vi "SVT Exp Avg Sound Level (1 Ch).vi"(6 "restart averaging (F)":bool, 8 "error in (no error)":errorcluster, 9 "time constant [ms]":dbl=125.0 format="%.2f", 10 "exponential mode":enum16{"Slow", "Fast", "Impulse", "Custom"}(ring)=enum."Fast", 11 "scaled signal [EU]":waveform(dbl)) -> (0 "error out":errorcluster, 1 "actual time constant [ms]":dbl=nan format="%.2f", 2 "unit label":string, 3 "exp avg sound level [dB EU]":waveform(dbl), 4 "maximum sound level [dB EU]":dbl=nan format="%.2f")   [LabVIEW 2017]
doc: "Computes the exponential averaged sound level of <B>scaled signal [EU]</B> based on <B>exponential mode</B> and returns the sound level for the signal in <B>exp avg sound level [dB EU]</B>. The SVL Exp Avg Sound Level VI returns the exponential average sound level computed after each individual sample of the time record. You can use this polymorphic VI to compute the exponential averaged sound level for a single channel or for N channels. The data type you wire to the <B>scaled signal [EU]</B> input determines the polymorphic instance to use."
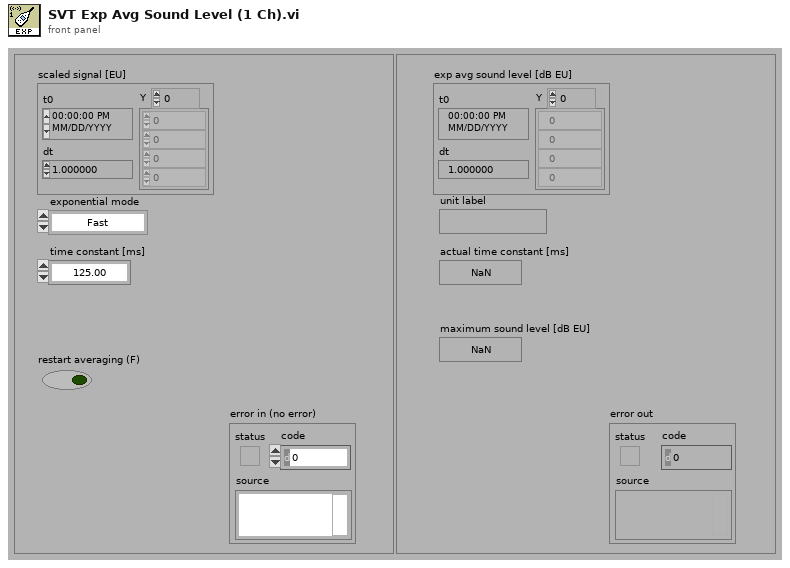
[diagram p1: front panel]
types:
  T1 = enum16{"RMS", "Running RMS", "Exp avg  ", "Dec exp avg ", "Peak", "Crest"}
  T2 = enum16{"Reset filter", "Restart averaging", "Continue processing"}
  T3 = typedef "svc_Channel Info.ctl" = cluster{"sensor sensitivity":dbl, "engineering units":T4, "dB reference":dbl, "custom label":string, "weighting filter":T5, "pregain":dbl}
  T4 = typedef "svc_Engineering Units Text Ring.ctl" = u16
  T5 = typedef "svc_Weighting Filter Text Ring.ctl" = u16
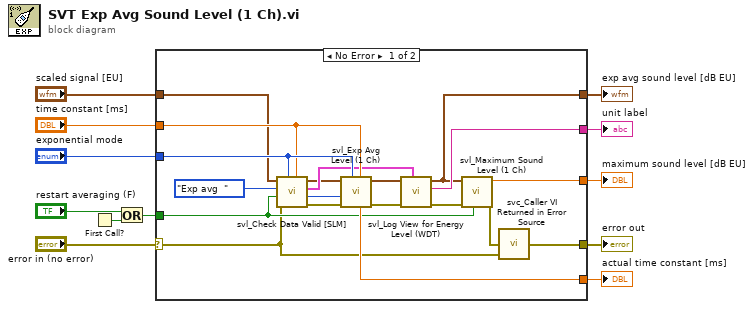
[diagram p0: block diagram]
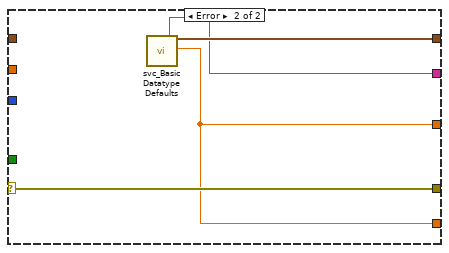
[diagram p2: hidden frame]
diagram:
  n1 = First Call?() -> (First Call?: T/F=w8:bool)
  n2 = Or(x="restart averaging (F)", y=w8) -> (x .or. y?=w7:bool)
  n3 = case shown="No Error" "error in (no error)" {
    tunnel: [w31 w33] -> w12
    tunnel: [w17 w34] -> w11
    tunnel: "scaled signal [EU]" -> [w16 _]
    tunnel: w7 -> [w20 _]
    tunnel: "exponential mode" -> [w27 _]
    tunnel: "time constant [ms]" -> [w26 _]
    tunnel: [w25 w32] -> w4
    tunnel: [w23 w35] -> w3
    selector: "error in (no error)" -> [w13 w35]
    tunnel: [w19 w32] -> w1
    frame No Error {
      n4 = call <vilib>:"svl_Check Data Valid [SLM].vi"("time constant [ms]"=w26, "exponential mode"=w27, "error in (no error)"=w13, "restart averaging (F)"=w20, "Level Analysis"=T1."Exp avg  ", "scaled signal [EU]"=w16) -> ("error out"=w28:errorcluster, "processing state"=w24:T2, "channel info"=w15:T3, "dup scaled signal [EU]"=w14:waveform(dbl))  [unwired: 2 in]
      n5 = call <vilib>:"svl_Exp Avg Level (1 Ch).vi"("timeConstant"=w26, "exponential mode"=w27, "error in (no error)"=w28, "processing state"=w24, "scaledSignal"=w14) -> ("error out"=w30:errorcluster, "scaledSignal"=w29:waveform(dbl), "actual time constant [ms]"=w25:dbl)  [unwired: 3 in, 1 out]
      n6 = call <vilib>:"svl_Log View for Energy Level (WDT).vi"("channel info"=w15, "error in (no error)"=w30, "scaledSignal"=w29) -> ("error out"=w22:errorcluster, "unit label"=w31:string, "scaledSignal"=w17:waveform(dbl))  [unwired: 6 in]
      n7 = call <vilib>:"svl_Maximum Sound Level (1 Ch).vi"("restart averaging (F)"=w20, "error in (no error)"=w22, "energy level [dB]"=w17) -> ("error out"=w21:errorcluster, "maximum sound level [dB EU]"=w19:dbl)  [unwired: 7 in]
      n8 = call <vilib>:"svc_Caller VI Returned in Error Source.vi"("warning input to caller"=w13, "error in (no error)"=w21) -> ("error out"=w23:errorcluster)  [unwired: 3 in]
    }
    frame Error {
      n9 = call <vilib>:"svc_Basic Datatype Defaults.vi"() -> ("empty string"=w33:string, "empty waveform"=w34:waveform(dbl), "NaN"=w32:dbl)  [unwired: 7 in, 10 out]
    }
  }
  "exp avg sound level [dB EU]" <- w11
  "actual time constant [ms]" <- w4
  "unit label" <- w12
  "error out" <- w3
  "maximum sound level [dB EU]" <- w1
